vi "PV ActiveLine - Display Resolution (TPG361).vi"(7 "W/R":bool, 8 "Fehler (Eingang)":errorcluster, 10 "Display control digits":i32(ring) items=["Auto (default)", "One digit", "Two digits", "Three digits", "Four digits"], 11 "Referenz in":refnum<visa-resource-name>) -> (0 "Cluster (Ausgang)":errorcluster, 2 "Get Display control digits":i32(ring) items=["Auto (default)", "One digit", "Two digits", "Three digits", "Four digits"], 3 "Referenz out":refnum<visa-resource-name>)   [LabVIEW 2013, in "PV ActiveLine.lvlib"]
doc: "DCD - Display Resolution\n\nTransmit: DCD [a]\nReceive: a\n\nResolution a =\n0 –> AUTO (default)\n1 –> One digit\n2 –> Two digits\n3 –> Three digits\n4 –> Four digits\n\nWhen the PrE is ON and the pressure is in the range p<1.0E-4 hPa the display resolution of the PCR Gauge is reduced by one decimal digit."
uses:
  <instrlib>/PV ActiveLine/PV ActiveLine.lvlib
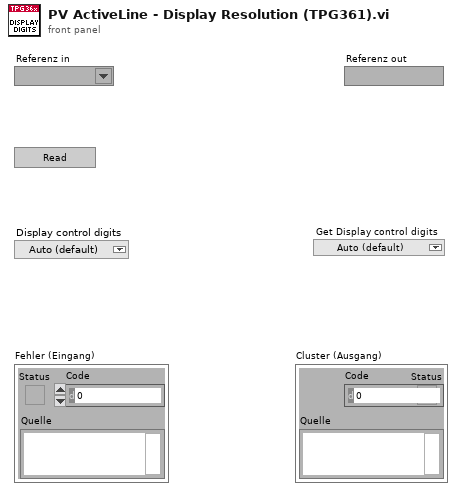
[diagram p1: front panel]
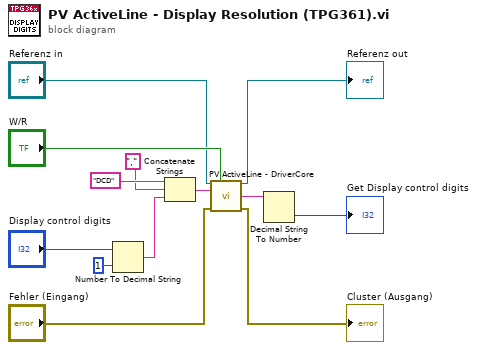
[diagram p0: block diagram]
diagram:
  n1 = Number To Decimal String(number="Display control digits", width (-)=i16 1) -> (decimal integer string=w11:string)
  n2 = Concatenate Strings("DCD" ("Command"), "," ("Command"), w11) -> (w7:string)
  n3 = call <instrlib>:"PV ActiveLine - DriverCore.vi"("Referenz in"="Referenz in", "Write/Read"="W/R", "Command"=w7, "Fehler (Eingang)"="Fehler (Eingang)") -> ("Referenz out"=→"Referenz out":refnum<visa-resource-name>, "String Out"=w9:string, "Cluster (Ausgang)"=→"Cluster (Ausgang)":errorcluster)  [unwired: 9 in]
  n4 = Decimal String To Number(string=w9) -> (number=→"Get Display control digits":i32)  [unwired: 2 in, 1 out]
